vi "SQL Time to Timestamp.vi"(1 "Get:Get String":string) -> (0 "Time Stamp":timestamp)   [LabVIEW 2019, in "Database Viewer.lvclass"]
uses:
  Database Viewer.lvclass
panel:
  out "error out":errorcluster
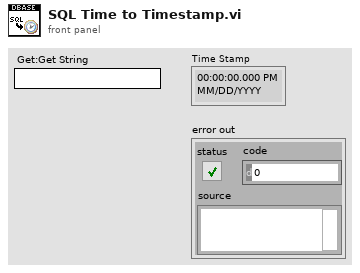
[diagram p1: front panel]
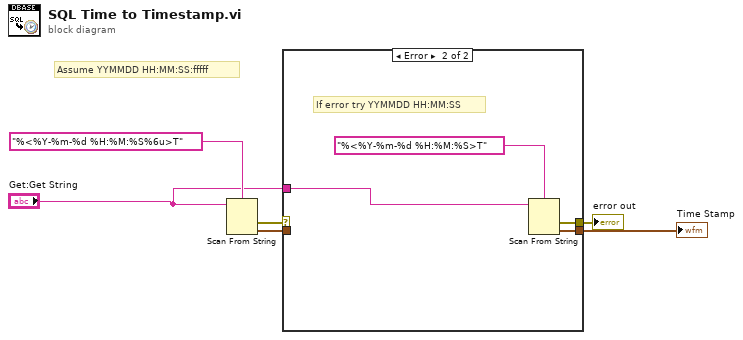
[diagram p0: block diagram]
diagram:
  # "Assume YYMMDD HH:MM:SS:fffff"
  n1 = Scan From String(format string="%<%Y-%m-%d %H:%M:%S%6u>T", input string="Get:Get String") -> (error out=w4:errorcluster, output 1=w2:timestamp)  [unwired: 3 in, 2 out]
  n2 = case shown="Error" w4 {
    selector: w4 -> [w7 _]
    tunnel: w2 -> [w8 _]
    tunnel: [w8 w9] -> w6
    tunnel: [w7 w11] -> w5
    tunnel: "Get:Get String" -> [_ w10]
    frame No Error {
    }
    frame Error {
      # "If error try YYMMDD HH:MM:SS"
      n3 = Scan From String(format string="%<%Y-%m-%d %H:%M:%S>T", input string=w10) -> (error out=w11:errorcluster, output 1=w9:timestamp)  [unwired: 3 in, 2 out]
    }
  }
  "error out" <- w5
  "Time Stamp" <- w6
